vi "EOL TM AW Formula.vi"(4 "Orifice (mm)":dbl=13.0, 7 "Suction Pressure (kPa)":dbl=20.0, 8 "error in (no error)":errorcluster, 9 "Ambient Pressure (kPa) Bt":dbl=105.0 format="%#_15g", 10 "Ambient Temperature (C)":dbl=25.0, 11 "Ambient Humudity (%)":dbl=60.0) -> (0 "error out":errorcluster, 2 "Flow-Rate (l/s), Q":dbl, 3 "Suction Power in Air Watt":dbl)   [LabVIEW 2017]
panel:
  out "Flow coefficient K1":dbl
  out "Corrected Suction (kPa), Hs":dbl
  out "Density Ratio, Dr":dbl
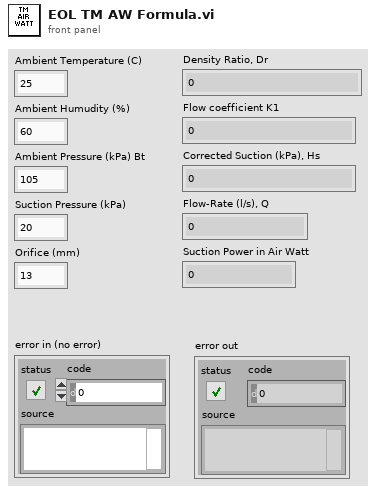
[diagram p1: front panel]
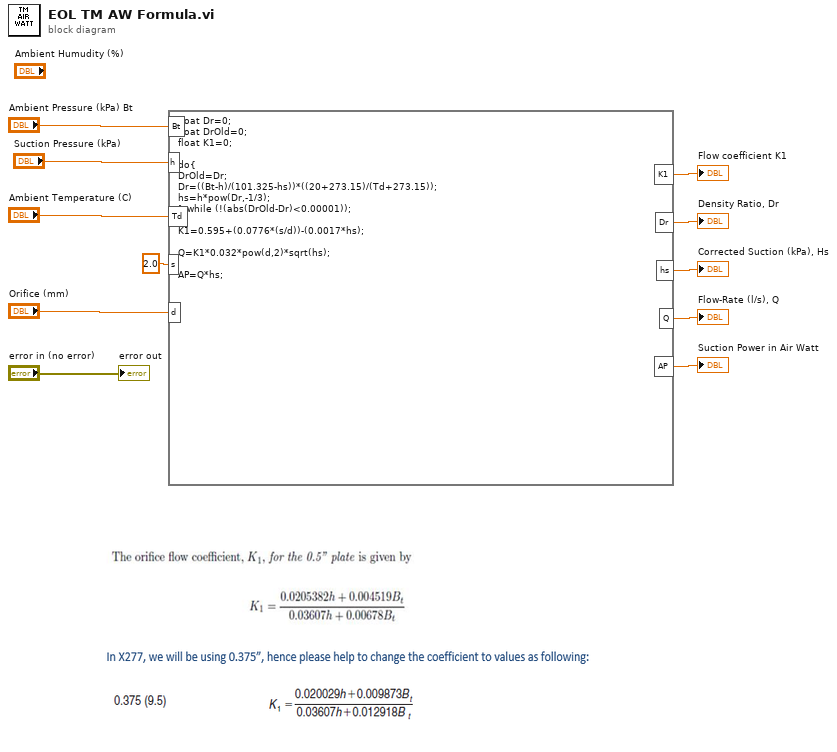
[diagram p0: block diagram]
diagram:
  n1 = formula code="float Dr=0;\nfloat DrOld=0;\nfloat K1=0;\n\ndo{\nDrOld=Dr;\nDr=((Bt-h)/(101.325-hs))*((20+273.15)/(Td+273.15));\nhs=h*pow(Dr,-1/3);\n} while (!(abs(DrOld-Dr)<0.00001));\n\nK1=0.595+(0.0776*(s/d))-(0.0017*hs);\n\nQ=K1*0.032*pow(d,2)*sqrt(hs);\n\nAP=Q*hs;"("s"=2.0 ("input variable"), "Td"="Ambient Temperature (C)", "Bt"="Ambient Pressure (kPa) Bt", "h"="Suction Pressure (kPa)", "d"="Orifice (mm)") -> ("Dr"=→"Density Ratio, Dr":dbl, "hs"=→"Corrected Suction (kPa), Hs":dbl, "K1"=→"Flow coefficient K1":dbl, "Q"=→"Flow-Rate (l/s), Q":dbl, "AP"=→"Suction Power in Air Watt":dbl)
  "error out" <- "error in (no error)"
